vi "DAQ_TTR Meas Configure and Measure.vi"(0 "DAQmx Task In":refnum<k21>, 2 "Execution Option":T7, 5 "Range and Terminal Settings":T1={"Global Settings"={"Min Temp (degC)"=0.0, "Max Temp (degC)"=100.0, "Vex Value (V)"=5.0, "R1 (Ohm)"=1000.0, "Terminal Configuration"=10083, "Thermistor Parameters"={"Type"=enum."A B C", "ABC Parameters"={"A"=0.0, "B"=0.0, "C"=0.0}, "Beta Parameters"={"Beta Value (K)"=0.0, "R0 (Ohm)"=0.0}}}, "Specific Channel Settings"=[]} {"Specific Channel Settings"."Terminal Configuration" items=["RSE"=10083, "NRSE"=10078, "Differential"=10106]; "Specific Channel Settings"."Thermistor Parameters"."Beta Parameters"."R0 (Ohm)" format="%#.6p"; "Specific Channel Settings"."Thermistor Parameters"."Beta Parameters"."Beta Value (K)" format="%.2f"; "Specific Channel Settings"."Thermistor Parameters"."ABC Parameters"."C" format="%^.6e"; "Specific Channel Settings"."Thermistor Parameters"."ABC Parameters"."B" format="%^.6e"; "Specific Channel Settings"."Thermistor Parameters"."ABC Parameters"."A" format="%^.6e"; "Specific Channel Settings"."R1 (Ohm)" format="%#.2p"; "Specific Channel Settings"."Vex Value (V)" format="%#.2p"; "Specific Channel Settings"."Max Temp (degC)" format="%.2f"; "Specific Channel Settings"."Min Temp (degC)" format="%.2f"; "Global Settings"."Terminal Configuration" items=["RSE"=10083, "NRSE"=10078, "Differential"=10106]; "Global Settings"."Thermistor Parameters"."Beta Parameters"."R0 (Ohm)" format="%#.6p"; "Global Settings"."Thermistor Parameters"."Beta Parameters"."Beta Value (K)" format="%.2p"; "Global Settings"."Thermistor Parameters"."ABC Parameters"."C" format="%^.6e"; "Global Settings"."Thermistor Parameters"."ABC Parameters"."B" format="%^.6e"; "Global Settings"."Thermistor Parameters"."ABC Parameters"."A" format="%^.6e"; "Global Settings"."R1 (Ohm)" format="%#.2p"; "Global Settings"."Vex Value (V)" format="%#.2f"; "Global Settings"."Max Temp (degC)" format="%.2f"; "Global Settings"."Min Temp (degC)" format="%.2f"}, 7 "Timing and Trigger Settings":T8={"Timing Settings"={"Sample Clock Source"="OnboardClock", "Sample Rate(Hz)"=10000.0, "Number of Samples"=1000, "Sample Timing Engine"=enum."Auto"}, "Trigger Settings"={"Trigger Type"=enum."No Trigger", "Digital Start Trigger Source"="", "Digital Start Trigger Edge"=10280}} {"Trigger Settings"."Digital Start Trigger Edge" items=["Rising"=10280, "Falling"=10171]; "Timing Settings"."Sample Rate(Hz)" format="%.2p"}, 11 "error in":errorcluster) -> (4 "DAQmx Task Out":refnum<k21>, 6 "Temperature Waveforms":waveform(dbl)[](graph), 8 "Temperature Measurements":T6 {"Averaged Temperature (K)" format="%.2p"; "Averaged Temperature (degC)" format="%.2p"}, 10 "Acquisition Time (s)":dbl format="%.2p", 15 "error out":errorcluster)   [LabVIEW 2021, in "DAQ_Temperature Thermistor Measurement.lvlib"]
doc: "Configure, initiate and fetch temperature measurements from the channels configured."
uses:
  DAQ_Temperature Thermistor Measurement.lvlib
  Typedefs/Timing & Trigger Settings.ctl
  Typedefs/Timing Settings.ctl
  Typedefs/Trigger Settings.ctl
  Common/Typedefs/Execution Options - Measure.ctl
  Typedefs/Temperature Thermistor Measurements.ctl
  Typedefs/Range and Terminal Settings.ctl
  Typedefs/Thermistor Parameters.ctl
  Typedefs/ABC Parameters.ctl
  Typedefs/Beta Parameters.ctl
  Typedefs/Specific Channel Settings.ctl
  <vilib>/DAQmx/read.llb/DAQmx Read (Analog 1D Wfm NChan NSamp).vi
  <vilib>/DAQmx/configure/timing.llb/DAQmx Timing (Sample Clock).vi
  <vilib>/DAQmx/configure/trigger.llb/DAQmx Start Trigger (Digital Edge).vi
  <vilib>/DAQmx/miscellaneous.llb/DAQmx Fill In Error Info.vi
  <resource>/objmgr/daqmx.rc
panel:
  # "Outputs"
  # "Inputs"
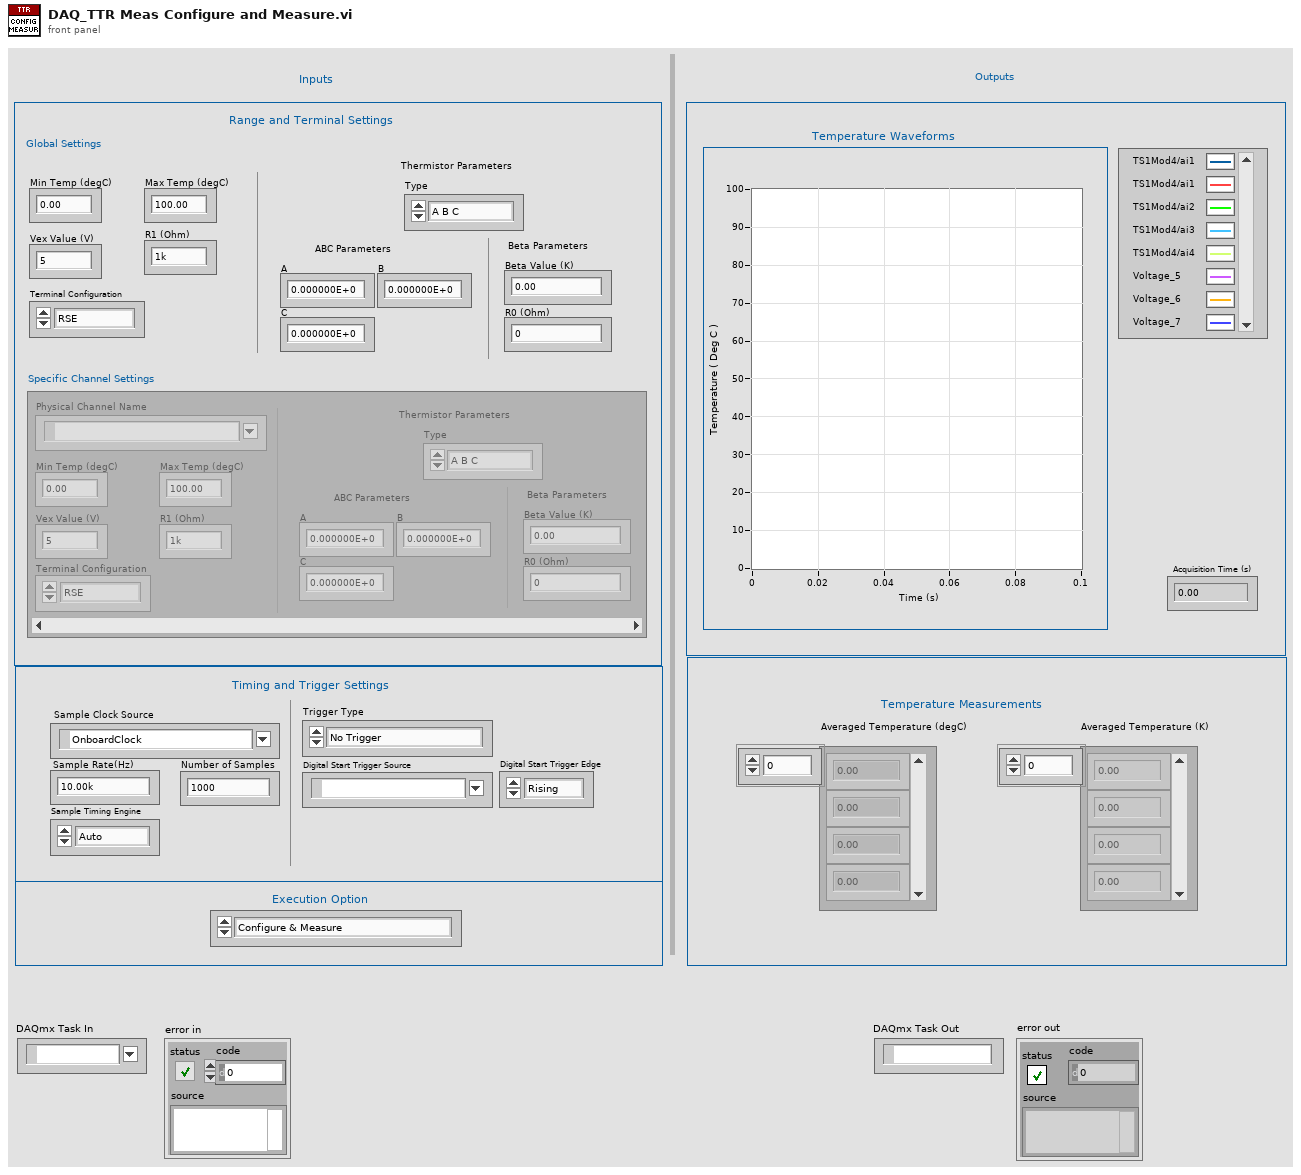
[diagram p1: front panel]
types:
  T1 = typedef "DAQ_Temperature Thermistor Measurement.lvlib/Range and Terminal Settings.ctl" = cluster{"Global Settings":cluster{"Min Temp (degC)":dbl, "Max Temp (degC)":dbl, "Vex Value (V)":dbl, "R1 (Ohm)":dbl, "Terminal Configuration":i32, "Thermistor Parameters":T2}, "Specific Channel Settings":T5[]}
  T2 = typedef "DAQ_Temperature Thermistor Measurement.lvlib/Thermistor Parameters.ctl" = cluster{"Type":enum16{"A B C", "Beta"}, "ABC Parameters":T3, "Beta Parameters":T4}
  T3 = typedef "DAQ_Temperature Thermistor Measurement.lvlib/ABC Parameters.ctl" = cluster{"A":dbl, "B":dbl, "C":dbl}
  T4 = typedef "DAQ_Temperature Thermistor Measurement.lvlib/Beta Parameters.ctl" = cluster{"Beta Value (K)":dbl, "R0 (Ohm)":dbl}
  T5 = typedef "DAQ_Temperature Thermistor Measurement.lvlib/Specific Channel Settings.ctl" = cluster{"Physical Channel Name":tag, "Min Temp (degC)":dbl, "Max Temp (degC)":dbl, "Vex Value (V) ":dbl, "R1 (Ohm)":dbl, "Terminal Configuration":i32, "Thermistor Parameters":T2}
  T6 = typedef "DAQ_Temperature Thermistor Measurement.lvlib/Temperature Thermistor Measurements.ctl" = cluster{"Averaged Temperature (degC)":dbl[], "Averaged Temperature (K)":dbl[]}
  T7 = typedef "Execution Options - Measure.ctl" = enum16{"Configure & Measure", "Configure only", "Measure only"}
  T8 = typedef "DAQ_Temperature Thermistor Measurement.lvlib/Timing & Trigger Settings.ctl" = cluster{"Timing Settings":T9, "Trigger Settings":T10}
  T9 = typedef "DAQ_Temperature Thermistor Measurement.lvlib/Timing Settings.ctl" = cluster{"Sample Clock Source":tag, "Sample Rate(Hz)":dbl, "Number of Samples":i32, "Sample Timing Engine":enum16{"te0", "te1", "ai", "Auto"}}
  T10 = typedef "DAQ_Temperature Thermistor Measurement.lvlib/Trigger Settings.ctl" = cluster{"Trigger Type":enum16{"No Trigger", "Digital Start"}, "Digital Start Trigger Source":tag, "Digital Start Trigger Edge":i32}
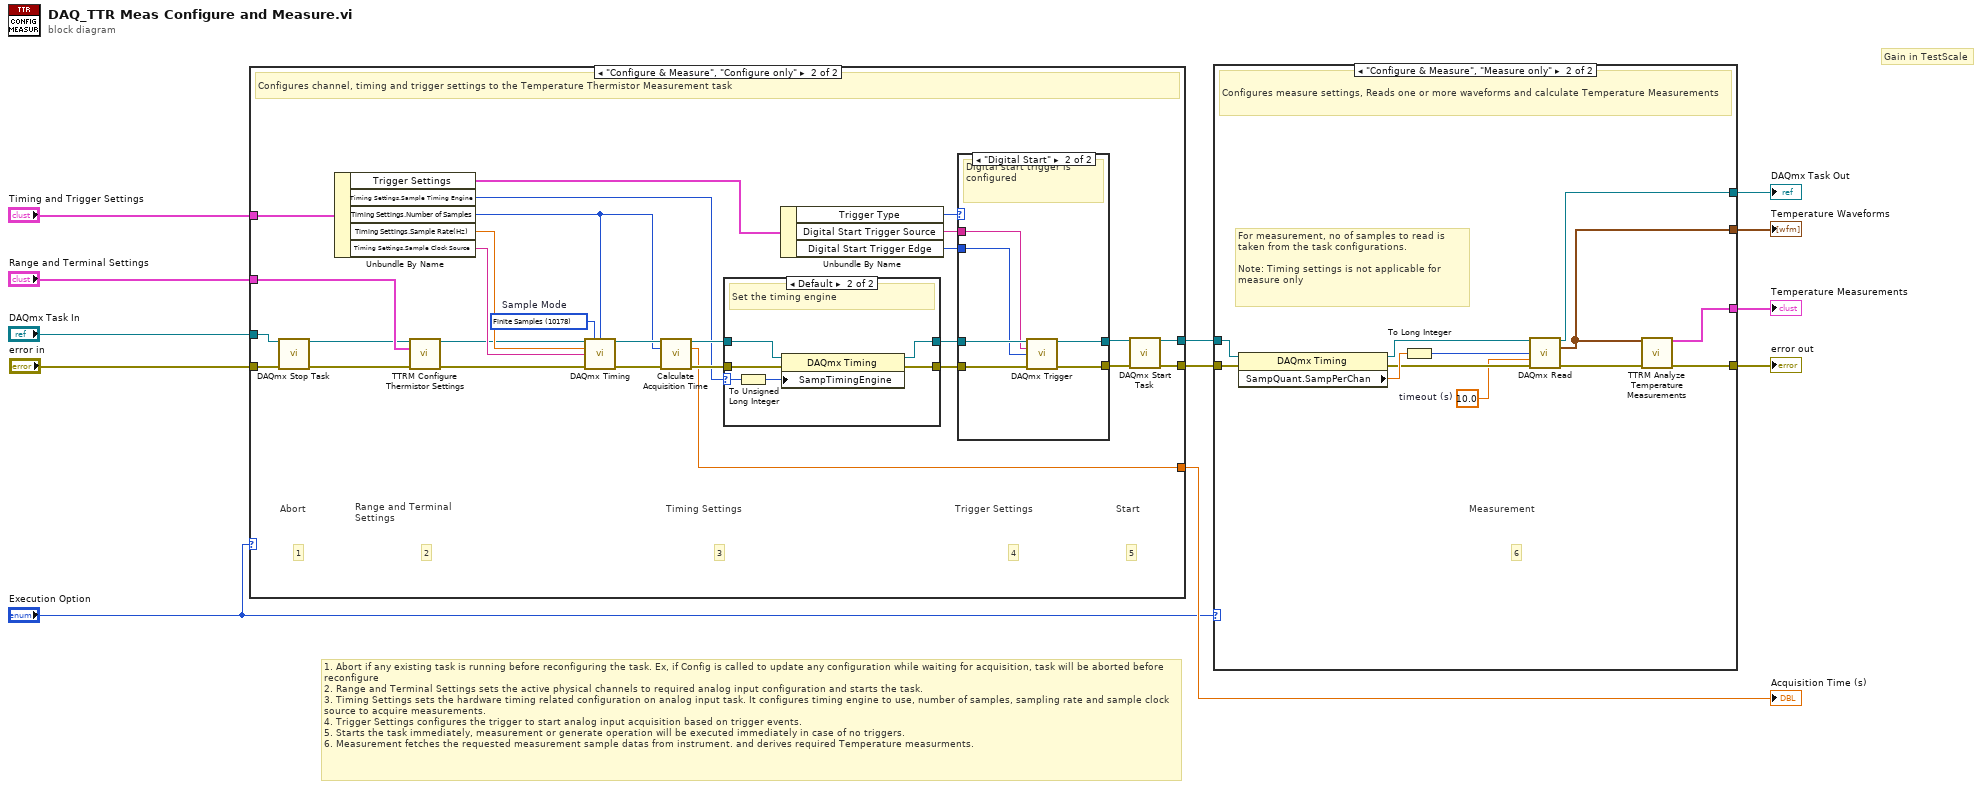
[diagram p0: block diagram]
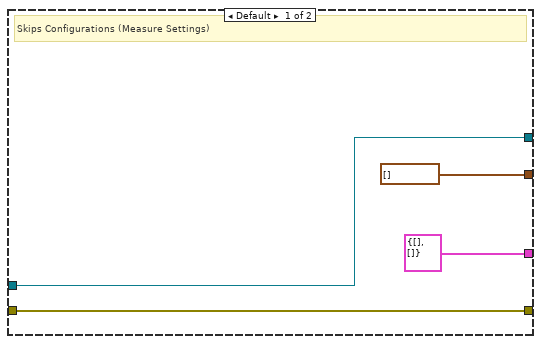
[diagram p5: hidden frame]
diagram:
  # "Gain in TestScale"
  # "1. Abort if any existing task is running before reconfiguring the task. Ex, if Config is called to update any configuration while waiting for acquisition, task will be aborted before reconfigure\n2. Range and Terminal Settings sets the active physical channels to required analog input configuration and starts the task.\n3. Timing Settings sets the hardware timing related configuration on analog input task. It configures timing engine to use, number of samples, sampling rate and sample clock source to acquire measurements.\n4. Trigger Settings configures the trigger to start analog input acquisition based on trigger events.\n5. Starts the task immediately, measurement or generate operation will be executed immediately in case of no triggers.\n6. Measurement fetches the requested measurement sample datas from instrument. and derives required Temperature measurments."
  n1 = case shown="\"Configure & Measure\", \"Configure only\"" "Execution Option" {
    tunnel: "error in" -> [w14 w19]
    tunnel: "DAQmx Task In" -> [w13 w20]
    tunnel: "Timing and Trigger Settings" -> [_ w36]
    tunnel: [w13 w17] -> w11
    tunnel: [w14 w30] -> w12
    tunnel: "Range and Terminal Settings" -> [_ w23]
    tunnel: [_ w16] -> w4
    frame Default {
      # "Skips Configurations (Channel, Timing and Trigger Settings)"
    }
    frame "Configure & Measure", "Configure only" {
      w40 = 10178 items=["Finite Samples"=10178, "Continuous Samples"=10123, "Hardware Timed Single Point"=12522]  # Sample Mode
      # "1"
      # "Abort"
      # "5"
      # "Start"
      # "4"
      # "3"
      # "2"
      # "Range and Terminal \nSettings"
      # "Trigger Settings"
      # "Timing Settings"
      # "Configures channel, timing and trigger settings to the Temperature Thermistor Measurement task"
      n2 = call <vilib>:"DAQmx Stop Task.vi"("task/channels in"=w20, "error in"=w19) -> ("task out"=w21:refnum<k21>, "error out"=w15:errorcluster)  [unwired: 12 in]
      n3 = Unbundle By Name(w36) -> ("Trigger Settings"=w22:T10, "Timing Settings.Sample Timing Engine"=w31:enum16{"te0", "te1", "ai", "Auto"}, "Timing Settings.Number of Samples"=w29:i32, "Timing Settings.Sample Rate(Hz)"=w37:dbl, "Timing Settings.Sample Clock Source"=w38:tag)
      n4 = call "TTRM Configure Thermistor Settings.vi"("DAQmx Task In"=w21, "Range and Terminal Settings"=w23, "error in (no error)"=w15) -> ("DAQmx Task Out"=w24:refnum<k21>, "error out"=w25:errorcluster)  [unwired: 11 in]
      n5 = call-poly <vilib>:"DAQmx Timing.vi"("task/channels in"=w24, "sample mode"=w40, "samples per channel"=w29, "rate"=w37, "source"=w38, "error in"=w25) -> ("task out"=w42:refnum<k21>, "error out"=w41:errorcluster)  [unwired: 8 in]
      n6 = call "Calculate Acquisition Time.vi"("Refnum in"=w42, "Number of Samples"=w29, "error in (no error)"=w41) -> ("Refnum out"=w33:refnum<k21>, "Acquisition Time Period (s)"=w16:dbl, "error out"=w39:errorcluster)  [unwired: 10 in]
      n7 = case shown="Default" w31 {
        selector: w31 -> [_ w46]
        tunnel: w39 -> [w44 w50]
        tunnel: [w44 w49] -> w34
        tunnel: w33 -> [w43 w48]
        tunnel: [w43 w47] -> w32
        frame "Auto" {
          # "Timing engine is auto-selected"
        }
        frame Default {
          # "Set the timing engine"
          n8 = To Unsigned Long Integer(number=w46) -> (unsigned 32bit integer=w45:u32)
          n9 = property class="DAQmx Timing"(reference=w48, error in=w50, "SampTimingEngine"=w45) -> (reference out=w47:refnum<k21>, error out=w49:errorcluster)
        }
      }
      n10 = Unbundle By Name(w22) -> ("Trigger Type"=w26:enum16{"No Trigger", "Digital Start"}, "Digital Start Trigger Source"=w28:tag, "Digital Start Trigger Edge"=w27:i32)
      n11 = case shown="\"Digital Start\"" w26 {
        tunnel: w32 -> [w52 w58]
        tunnel: w34 -> [w51 w57]
        tunnel: [w52 w56] -> w18
        tunnel: [w51 w55] -> w35
        tunnel: w28 -> [_ w54]
        tunnel: w27 -> [_ w53]
        frame Default {
          # "No Trigger settings has been configured"
        }
        frame "Digital Start" {
          # "Digital start trigger is configured"
          n12 = call-poly <vilib>:"DAQmx Trigger.vi"("task/channels in"=w58, "source"=w54, "edge"=w53, "error in"=w57) -> ("task out"=w56:refnum<k21>, "error out"=w55:errorcluster)  [unwired: 10 in]
        }
      }
      n13 = call <vilib>:"DAQmx Start Task.vi"("task/channels in"=w18, "error in"=w35) -> ("task out"=w17:refnum<k21>, "error out"=w30:errorcluster)  [unwired: 12 in]
    }
  }
  "Acquisition Time (s)" <- w4
  n14 = case shown="\"Configure & Measure\", \"Measure only\"" "Execution Option" {
    tunnel: w11 -> [w62 w70]
    tunnel: w12 -> [w61 w67]
    tunnel: [w62 w72] -> w10
    tunnel: [w61 w74] -> w8
    tunnel: [T6 {"Averaged Temperature (degC)"=[], "Averaged Temperature (K)"=[]} ("DC Measurements") w65] -> w2
    tunnel: [waveform(dbl)[] [] ("data") w64] -> w5
    frame Default {
      # "Skips Configurations (Measure Settings)"
    }
    frame "Configure & Measure", "Measure only" {
      w63 = 10.0  # timeout (s)
      # "For measurement, no of samples to read is taken from the task configurations.\n\nNote: Timing settings is not applicable for measure only"
      # "6"
      # "Measurement"
      # "Configures measure settings, Reads one or more waveforms and calculate Temperature Measurements"
      n15 = property class="DAQmx Timing"(reference=w70, error in=w67) -> (reference out=w71:refnum<k21>, error out=w68:errorcluster, "SampQuant.SampPerChan"=w69:dbl)
      n16 = To Long Integer(number=w69) -> (32bit integer=w66:i32)
      n17 = call-poly <vilib>:"DAQmx Read.vi"("task/channels in"=w71, "number of samples per channel"=w66, "timeout"=w63, "error in"=w68) -> ("task out"=w72:refnum<k21>, "data"=w64:waveform(dbl)[], "error out"=w73:errorcluster)  [unwired: 9 in]
      n18 = call "TTRM Analyze Temperature Measurements.vi"("Temperature Waveforms In"=w64, "error in (no error)"=w73) -> ("Temperature Measurements Out"=w65:T6, "error out"=w74:errorcluster)  [unwired: 12 in]
    }
  }
  "error out" <- w8
  "DAQmx Task Out" <- w10
  "Temperature Waveforms" <- w5
  "Temperature Measurements" <- w2
